vi "Utility Parse Binary String.vi"(10 "Input Binary String":string) -> (2 "Output Array":i16[](array[numeric]))   [LabVIEW 2014, in "Agilent ESG Series.lvlib"]
doc: "This VI parse binary string from instrument into output array.\n\nBinary string:\n\n#ABC\n\nA the number of decimal digits to follow in B.\nB a decimal number specifying the number of data bytes in C.\nC the binary waveform data."
uses:
  Agilent ESG Series.lvlib
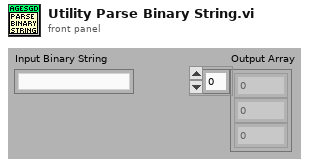
[diagram p1: front panel]
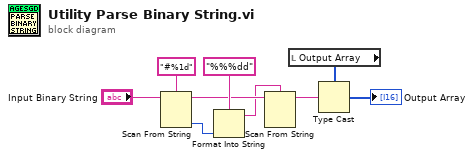
[diagram p0: block diagram]
diagram:
  n1 = Scan From String(format string="#%1d", input string="Input Binary String") -> (remaining string=w5:string, output 1=w7:i32)  [unwired: 3 in, 2 out]
  n2 = Format Into String(format string="%%%dd", w7) -> (resulting string=w4:string)  [unwired: 2 in, 1 out]
  n3 = Scan From String(format string=w4, input string=w5) -> (remaining string=w3:string)  [unwired: 4 in, 2 out]
  n4 = local read "Output Array"() -> (w1:i16[])
  n5 = Type Cast(type=w1, x=w3) -> (*(type *) &x=→"Output Array":i16[])
